vi "lock-in_send_order.vi"(6 "frequency (Hz)":sgl, 7 "inhibate?":bool=TRUE, 8 "amplitude":sgl format="%.14g", 9 "Chanel (cl)":cluster{"panel LI":u8, "channel LI":u8}, 10 "order":T2(ring), 11 "FPGA VI Reference In":T1) -> ()   [LabVIEW 2013]
uses:
  fpga-bitfile-ref.ctl
panel:
  out "order to send":u64
  out "(hi.lo)":u16
  out "(hi.lo) 2":u32
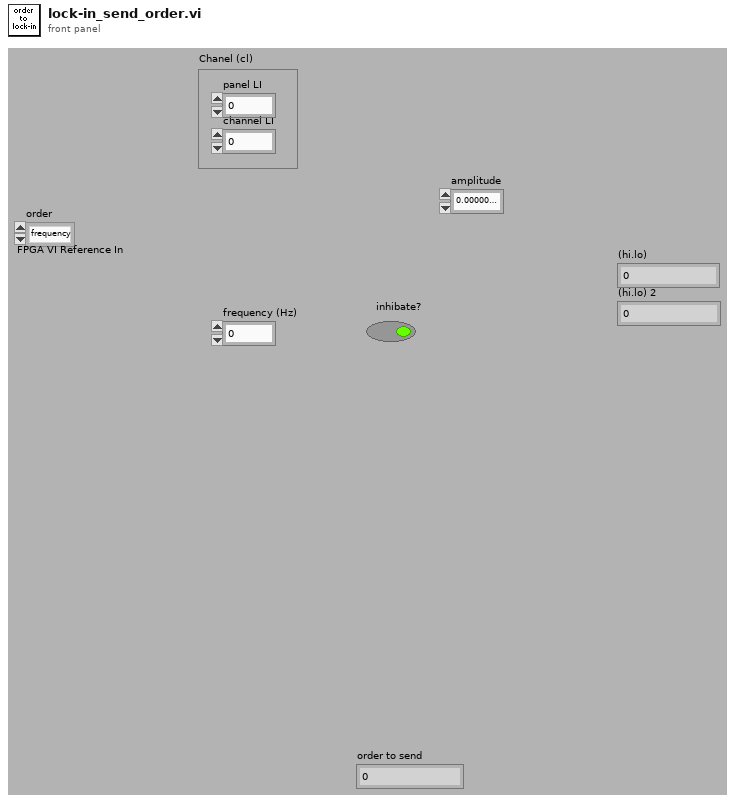
[diagram p1: front panel]
types:
  T1 = typedef "fpga-bitfile-ref.ctl" = refnum<k20>
  T2 = enum16{"frequency", "channel", "amplitude", "inhibate"}
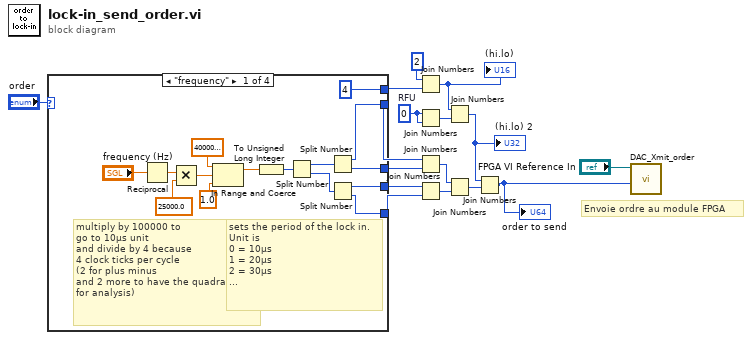
[diagram p0: block diagram]
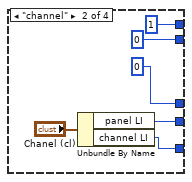
[diagram p2: hidden frame]
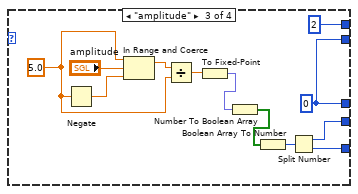
[diagram p3: hidden frame]
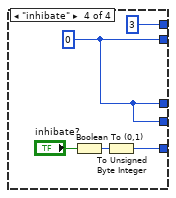
[diagram p4: hidden frame]
diagram:
  w14 = u8 0  # RFU
  # "Envoie ordre au module FPGA"
  n1 = case shown="\"frequency\"" "order" {
    tunnel: [w29 w33 w49 w51] -> w11
    tunnel: [w28 w32 w48 w54] -> w10
    tunnel: [w27 u8 0 w47 w54] -> w12
    tunnel: [w26 u8 0 w47 w54] -> w13
    tunnel: [u8 4 u8 1 u8 2 u8 3] -> w4
    frame "frequency" {
      # "multiply by 100000 to\ngo to 10µs unit\nand divide by 4 because\n4 clock ticks per cycle\n(2 for plus minus\nand 2 more to have the quadrature\nfor analysis)"
      # "sets the period of the lock in.\nUnit is\n0 = 10µs\n1 = 20µs\n2 = 30µs\n..."
      n2 = Reciprocal(x="frequency (Hz)") -> (1/x=w23:sgl)
      n3 = Multiply(x=w23, y=sgl 25000.0) -> (x*y=w21:sgl)
      n4 = In Range and Coerce(upper limit=sgl 4000000000.0 ("limite inférieure"), x=w21, lower limit=sgl 1.0 ("limite inférieure")) -> (coerced(x)=w18:sgl)  [unwired: 1 out]
      n5 = To Unsigned Long Integer(number=w18) -> (unsigned 32bit integer=w17:u32)
      n6 = Split Number(x=w17) -> (hi(x)=w30:u16, lo(x)=w31:u16)
      n7 = Split Number(x=w30) -> (hi(x)=w26:u8, lo(x)=w27:u8)
      n8 = Split Number(x=w31) -> (hi(x)=w28:u8, lo(x)=w29:u8)
    }
    frame "channel" {
      n9 = Unbundle By Name("Chanel (cl)") -> ("panel LI"=w32:u8, "channel LI"=w33:u8)
    }
    frame "amplitude" {
      w40 = sgl 5.0 ("limite supérieure")
      w47 = u8 0
      n10 = Negate(x=w40) -> (-x=w44:sgl)
      n11 = In Range and Coerce(upper limit=w40, x="amplitude", lower limit=w44) -> (coerced(x)=w43:sgl)  [unwired: 1 out]
      n12 = Divide(x=w43, y=w40) -> (x/y=w42:sgl)
      n13 = To Fixed-Point ("En virgule fixe")(number=w42) -> (fixed-point=w39:fxp<+/-,16,1>)  [unwired: 1 out]
      n14 = Number To Boolean Array(number=w39) -> (Boolean array=w38:bool[])
      n15 = Boolean Array To Number ("Tableau de booléens en nombre")(Boolean array=w38) -> (number=w41:u16)
      n16 = Split Number(x=w41) -> (hi(x)=w48:u8, lo(x)=w49:u8)
    }
    frame "inhibate" {
      w54 = u8 0
      n17 = Boolean To (0,1)(Boolean="inhibate?") -> (0, 1=w52:i16)
      n18 = To Unsigned Byte Integer(number=w52) -> (unsigned 8bit integer=w51:u8)
    }
  }
  n19 = Join Numbers(hi=u8 2, lo=w4) -> ((hi.lo)=w6:u16)
  "(hi.lo)" <- w6
  n20 = Join Numbers(hi=w14, lo=w14) -> ((hi.lo)=w7:u16)
  n21 = Join Numbers(hi=w13, lo=w12) -> ((hi.lo)=w8:u16)
  n22 = Join Numbers(hi=w10, lo=w11) -> ((hi.lo)=w9:u16)
  n23 = Join Numbers(hi=w6, lo=w7) -> ((hi.lo)=w2:u32)
  "(hi.lo) 2" <- w2
  n24 = Join Numbers(hi=w8, lo=w9) -> ((hi.lo)=w3:u32)
  n25 = Join Numbers(hi=w2, lo=w3) -> ((hi.lo)=w16:u64)
  "order to send" <- w16
  n26 = call "DAC_Xmit_order.vi"("Order in"=w16, "FPGA VI Reference In"="FPGA VI Reference In") -> ()  [unwired: 10 out]
